vi "Read Force Setpoint.vi"(11 "StartOpenLoopScan in":refnum<class "StartOpenLoopScan.lvclass">) -> (2 "Force Setpoint":dbl[unit], 3 "StartOpenLoopScan out":refnum<class "StartOpenLoopScan.lvclass">)   [LabVIEW 2015]
uses:
  StartOpenLoopScan.lvclass
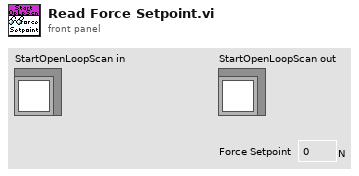
[diagram p1: front panel]
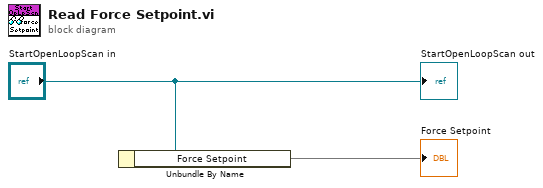
[diagram p0: block diagram]
diagram:
  n1 = Unbundle By Name("StartOpenLoopScan in") -> ("Force Setpoint"=→"Force Setpoint")
  "StartOpenLoopScan out" <- "StartOpenLoopScan in"
